vi "initial_guess.vi"(8 "Error In":errorcluster, 9 "Angle Guess Offset":dbl, 10 "Intensities":dbl[](array[numeric]), 11 "Angles":dbl[](array[numeric])) -> (0 "Error Out":errorcluster, 3 "Guess":dbl[](array[numeric]))   [LabVIEW 2019]
doc: "Creates the initial guess for the LM fitting of the angle/intensity curve."
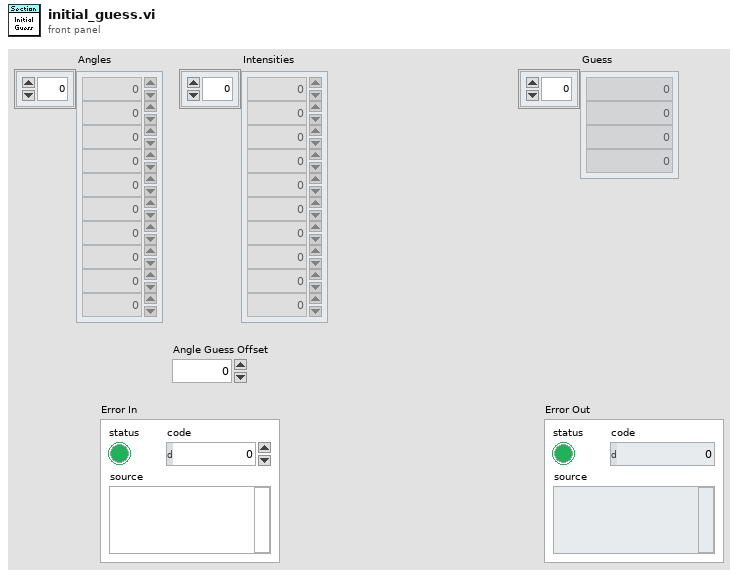
[diagram p1: front panel]
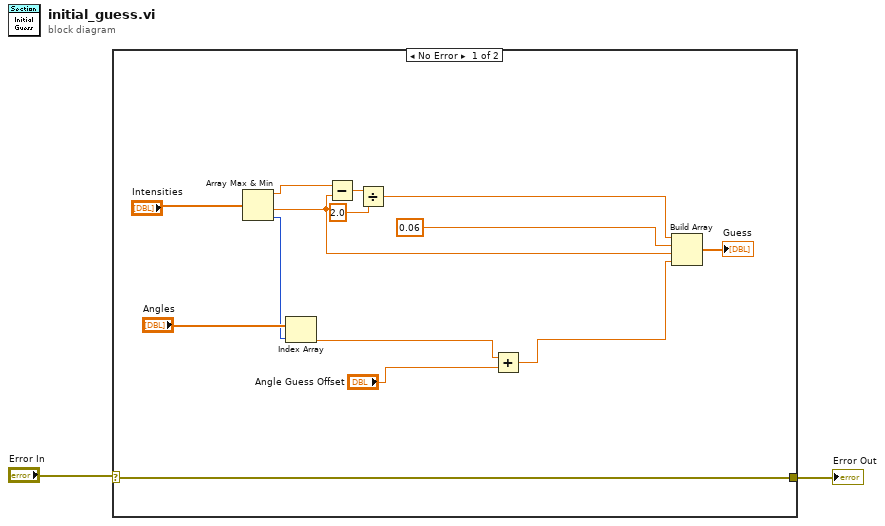
[diagram p0: block diagram]
diagram:
  n1 = case shown="No Error" "Error In" {
    selector: "Error In" -> [w10 w17]
    tunnel: [w10 w17] -> w1
    frame No Error {
      n2 = Array Max & Min(array="Intensities") -> (max value=w15:dbl, min value=w6:dbl, min index (indices)=w11:i32)  [unwired: 1 out]
      n3 = Index Array(array="Angles", index=w11) -> (element=w4:dbl)
      n4 = Subtract(x=w15, y=w6) -> (x-y=w14:dbl)
      n5 = Divide(x=w14, y=2.0) -> (x/y=w8:dbl)
      n6 = Add(x=w4, y="Angle Guess Offset") -> (x+y=w3:dbl)
      n7 = Build Array(w8, 0.06 ("B"), w6, w3) -> (→"Guess":dbl[])
    }
    frame Error {
    }
  }
  "Error Out" <- w1
